vi "pulse_generator_multiheater_refnum_switch_value_getter.vi"(0 "On/Off Refnums":refnum<vi>[](array[refnum]), 1 "Power Array":dbl[](array[numeric]) format="%#_13g") -> (2 "Analog[0-10]":dbl[](array[numeric]) format="%#_13g", 3 "Total Power":dbl, 4 "Digital":bool[](array[boolean]))   [LabVIEW 2017]
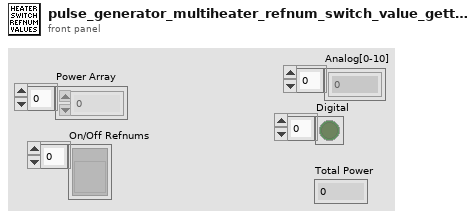
[diagram p1: front panel]
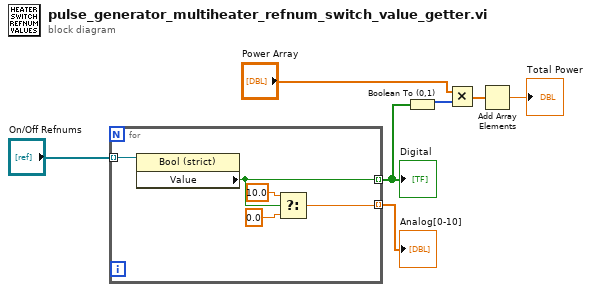
[diagram p0: block diagram]
diagram:
  n1 = for {
    tunnel: "On/Off Refnums" -> [w12] mode=indexing
    tunnel: [w9] -> w7 mode=indexing
    tunnel: [w8] -> w5 mode=indexing
    n2 = property class="Bool (strict)"(reference=w12) -> ("Value"=w8:bool)  [unwired: 1 in, 2 out]
    n3 = Select(t=10.0, s=w8, f=0.0) -> (s? t:f=w9:dbl)
  }
  "Analog[0-10]" <- w7
  "Digital" <- w5
  n4 = Boolean To (0,1)(Boolean=w5) -> (0, 1=w4:i16[])
  n5 = Multiply(x="Power Array", y=w4) -> (x*y=w2:dbl[])
  n6 = Add Array Elements(numeric array=w2) -> (sum=→"Total Power":dbl)
